vi "MainVI.vi"() -> ()   [LabVIEW 2026]
uses:
  <instrlib>/MicroPulse/Public/Data/Datatypes/TCP config.ctl
  <instrlib>/MicroPulse/Public/Data/Datatypes/MP - pulser voltage.ctl
  <instrlib>/MicroPulse/Public/Data/Datatypes/MP - pulse damping.ctl
  <instrlib>/MicroPulse/Public/Data/Datatypes/MP - frequency filter.ctl
  <instrlib>/MicroPulse/Public/Data/Datatypes/MP - waveform type.ctl
  <instrlib>/MicroPulse/Public/Data/Datatypes/MP - data output format.ctl
  <instrlib>/MicroPulse/Public/Data/Datatypes/MP - amplitude reporting mode.ctl
  <instrlib>/MicroPulse/Public/Data/Datatypes/MP - averaging.ctl
  <instrlib>/MicroPulse/Public/Data/Datatypes/MP - echo gate mode.ctl
  <instrlib>/MicroPulse/MicroPulse_Driver.lvlib
panel:
  in  "stop":bool
  in  "Tab Control":T1(tab)
  in  "Calculated Diameter":T2
  in  "Calculate Scan":bool
  in  "Scan Information":T3
  in  "Scan Settings":T4
  in  "Channel Select Tab Control":enum32{"1", "2", "3", "4", "5", "6", "7"}(tab)
  in  "Damping":T5=enum."149W"
  in  "Flaw Gate (mm Ti)":T6
  in  "Backwall Gate (mm)":T7
  in  "Voltage":T8=enum."200V"
  in  "Width (ns)":u32=80
  in  "Smoothing":u16=1 caption="Smoothing (1-11)"
  in  "Filter":T9=enum."0.75-12MHz  Broadband"
  in  "Waveform Type":T10
  in  "A-Scan Window":cluster{"Start":dbl, "Range":dbl}={"Start"=0.0, "Range"=330.0}
  in  "C-Scan Collection":T11
  in  "Channel 1 Interface":T7
  in  "Gain (dB)":dbl=30.0 min=-6.0 max=70.0 step=0.25 format="%.2fdB"
  in  "Voltage 2":T8=enum."200V" caption="Voltage"
  in  "Damping 2":T5=enum."149W"
  in  "Width (ns)      2":u32=80
  in  "Gain (dB) 2":dbl=30.0 min=-6.0 max=70.0 step=0.25 format="%.2fdB"
  in  "Filter 2":T9=enum."0.75-12MHz  Broadband" caption="Filter"
  in  "Smoothing 2":u16=1 caption="Smoothing (1-11)"
  in  "Waveform Type 2":T10 caption="Waveform Type"
  in  "A-Scan Window 2":cluster{"Start":dbl, "Range":dbl}={"Start"=0.0, "Range"=330.0}
  out "Waveform Graph":u16[](graph)
  in  "Channel Select":string(combo)="1"
  in  "PRF":u16=50
  in  "MicroPulse Configuration":T12={"Connection ID"=refnum, "IP address"="10.1.1.2", "host port"=1067, "OC timeout"=-1, "Read timeout"=0, "Write timeout"=0} {"Write timeout" format="%dms"; "Read timeout" format="%dms"; "OC timeout" format="%dms"}
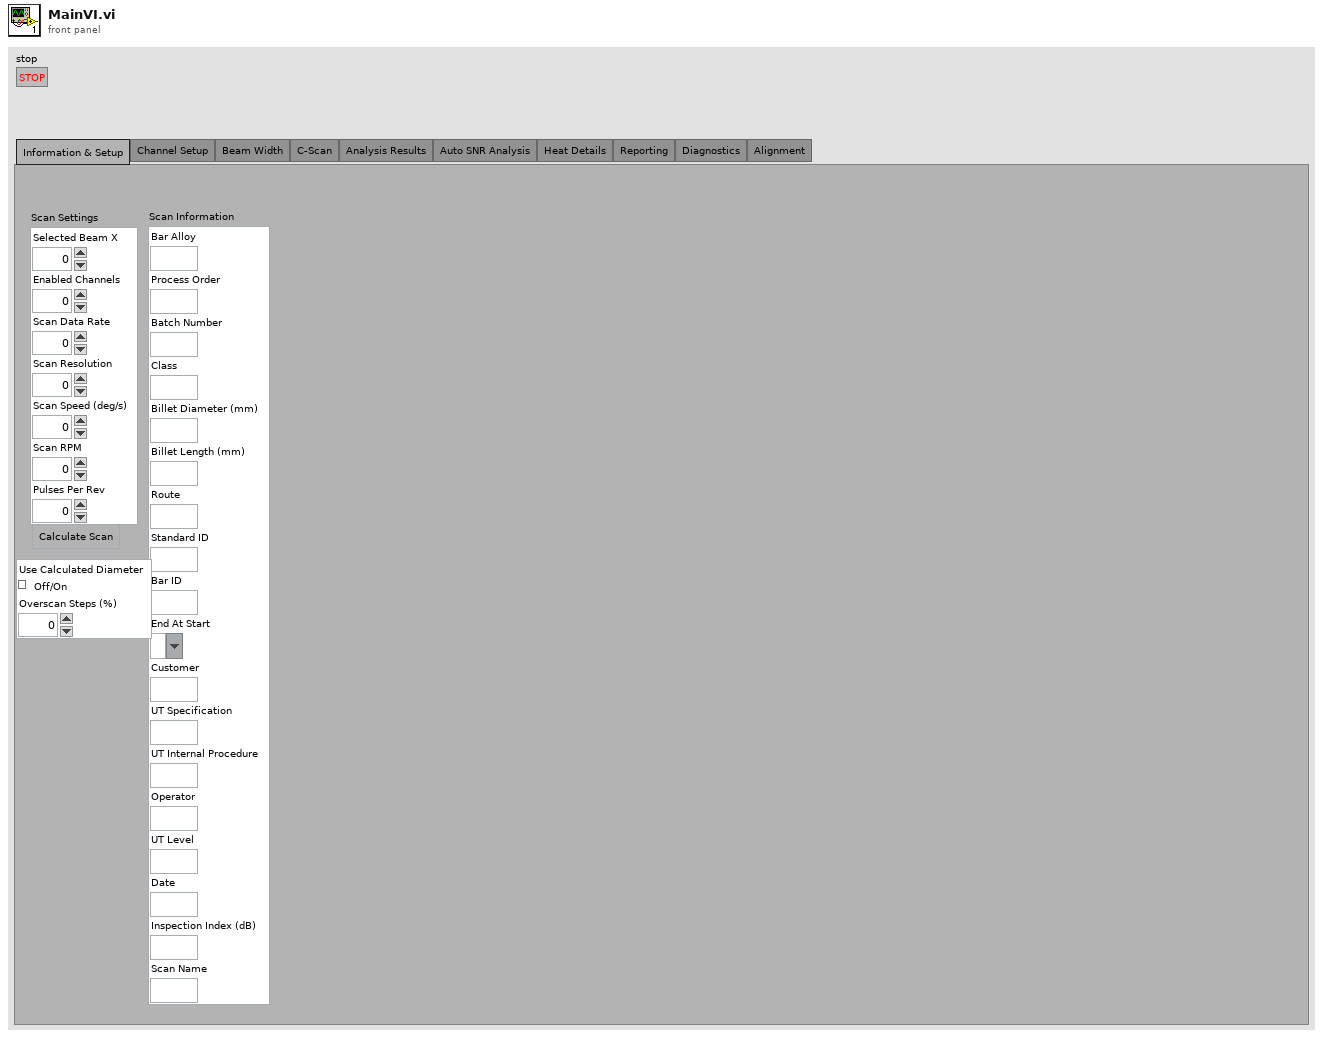
[diagram p1: front panel]
types:
  T1 = enum32{"Information & Setup", "Channel Setup", "Beam Width", "C-Scan", "Analysis Results", "Auto SNR Analysis", "Heat Details", "Reporting", "Diagnostics", "Alignment"}
  T2 = cluster{"Use Calculated Diameter":bool, "Overscan Steps (%)":dbl}
  T3 = cluster{"Bar Alloy":string, "Process Order":string, "Batch Number":string, "Class":string, "Billet Diameter (mm)":string, "Billet Length (mm)":string, "Route":string, "Standard ID":string, "Bar ID":string, "End At Start":string, "Customer":string, "UT Specification":string, "UT Internal Procedure":string, "Operator":string, "UT Level":string, "Date":string, "Inspection Index (dB)":string, "Scan Name":string}
  T4 = cluster{"Selected Beam X":dbl, "Enabled Channels":dbl, "Scan Data Rate":dbl, "Scan Resolution":dbl, "Scan Speed (deg/s)":dbl, "Scan RPM":dbl, "Pulses Per Rev":dbl}
  T5 = typedef "MicroPulse_Driver.lvlib/MP - pulse damping.ctl" = enum16{"660W", "458W", "220W", "149W", "102W", "82W", "63W", "51W"}
  T6 = cluster{"Start":dbl, "Length":dbl, "Threshold":dbl, "Water Path":dbl, "Gate Amplitude":dbl, "Gate TOF":dbl}
  T7 = cluster{"Start":dbl, "Length":dbl, "Threshold":dbl}
  T8 = typedef "MicroPulse_Driver.lvlib/MP - pulser voltage.ctl" = enum16{"50V", "100V", "150V", "200V", "250V", "300V"}
  T9 = typedef "MicroPulse_Driver.lvlib/MP - frequency filter.ctl" = enum16{"No change", "1MHz Bandpass", "2MHz Bandpass", "4MHz Bandpass", "5MHz Bandpass", "10MHz Bandpass", "2.5-18MHz Broadband", "0.75-12MHz  Broadband", "0.5MHz Bandpass", "5MHz 2nd Order TOFD", "10MHz 2nd Order TOFD", "3.0-25MHz Broadband", "3.0-30MHz Broadband"}
  T10 = typedef "MicroPulse_Driver.lvlib/MP - waveform type.ctl" = enum16{"Rectified Signal", "RF Signal", "+Half Wave", "-Half Wave"}
  T11 = cluster{"Flaw Gate Amplitude":bool, "Flaw Gate TOF":bool, "Backwall Gate Amplitude":bool, "Backwall Gate TOF":bool}
  T12 = typedef "MicroPulse_Driver.lvlib/TCP config.ctl" = cluster{"Connection ID":refnum<k5>, "IP address":string, "host port":u16, "OC timeout":i32, "Read timeout":i32, "Write timeout":i32}
  T13 = typedef "MicroPulse_Driver.lvlib/MP - data output format.ctl" = enum16{"", "8-bit Mode", "10-bit Mode", "12-bit Mode", "16-bit Mode", "8-bit Log Mode", "12-bit Packed Mode"}
  T14 = typedef "MicroPulse_Driver.lvlib/MP - echo gate mode.ctl" = enum16{"Echo Trigger OFF", "Echo Gate Display Mode", "Echo Trigger ON", "Multi Gate or FMC Mode", "Reserved", "PA - Echo Trigger ON"}
  T15 = typedef "MicroPulse_Driver.lvlib/MP - averaging.ctl" = enum16{"None", "2", "4", "8", "16", "32", "64", "128", "256"}
  T16 = typedef "MicroPulse_Driver.lvlib/MP - amplitude reporting mode.ctl" = enum16{"1st Peak in gate", "Maximum Peak in gate", "All Peaks", "Ascan Data", "1st Threshold Crossing Peak", "Ascan + Peaks", "All Peaks for Multigate", "Peaks + Ascan for Multigate", "Peaks + P_Ascan for Multigate", "Full Matrix Capture"}
  T17 = typedef "MicroPulse_Driver.lvlib/MP - scan data info.ctl" = cluster{"Message Header":u16, "Error Message":u16, "Test No.":u32, "Channel No.":u8, "Sweep No.":u32, "Gate No.":u32, "DOF":T13, "retain data":T18, "scan data":u16[], "scan length":i32, "scan index":i32, "peak data":cluster{"timebase":u16[], "data":u16[]}, "#peaks":i32, "PRF":dbl, "IP":cluster{"Axis No.":u8, "Location":u32, "MIP location":u32, "MIP?":bool}, "echo range":u16, "ETG":bool, "CAL 0 complete":bool, "Axis Positions":T19}
  T18 = typedef "MicroPulse_Driver.lvlib/MP - retain scan.ctl" = enum16{"None", "Ascan", "Peaks"}
  T19 = typedef "MicroPulse_Driver.lvlib/MP - axis positions (LLC).ctl" = cluster{"Axis 1":u32, "Axis 2":u32, "Axis 3":u32, "Axis 4":u32, "Status":u8}
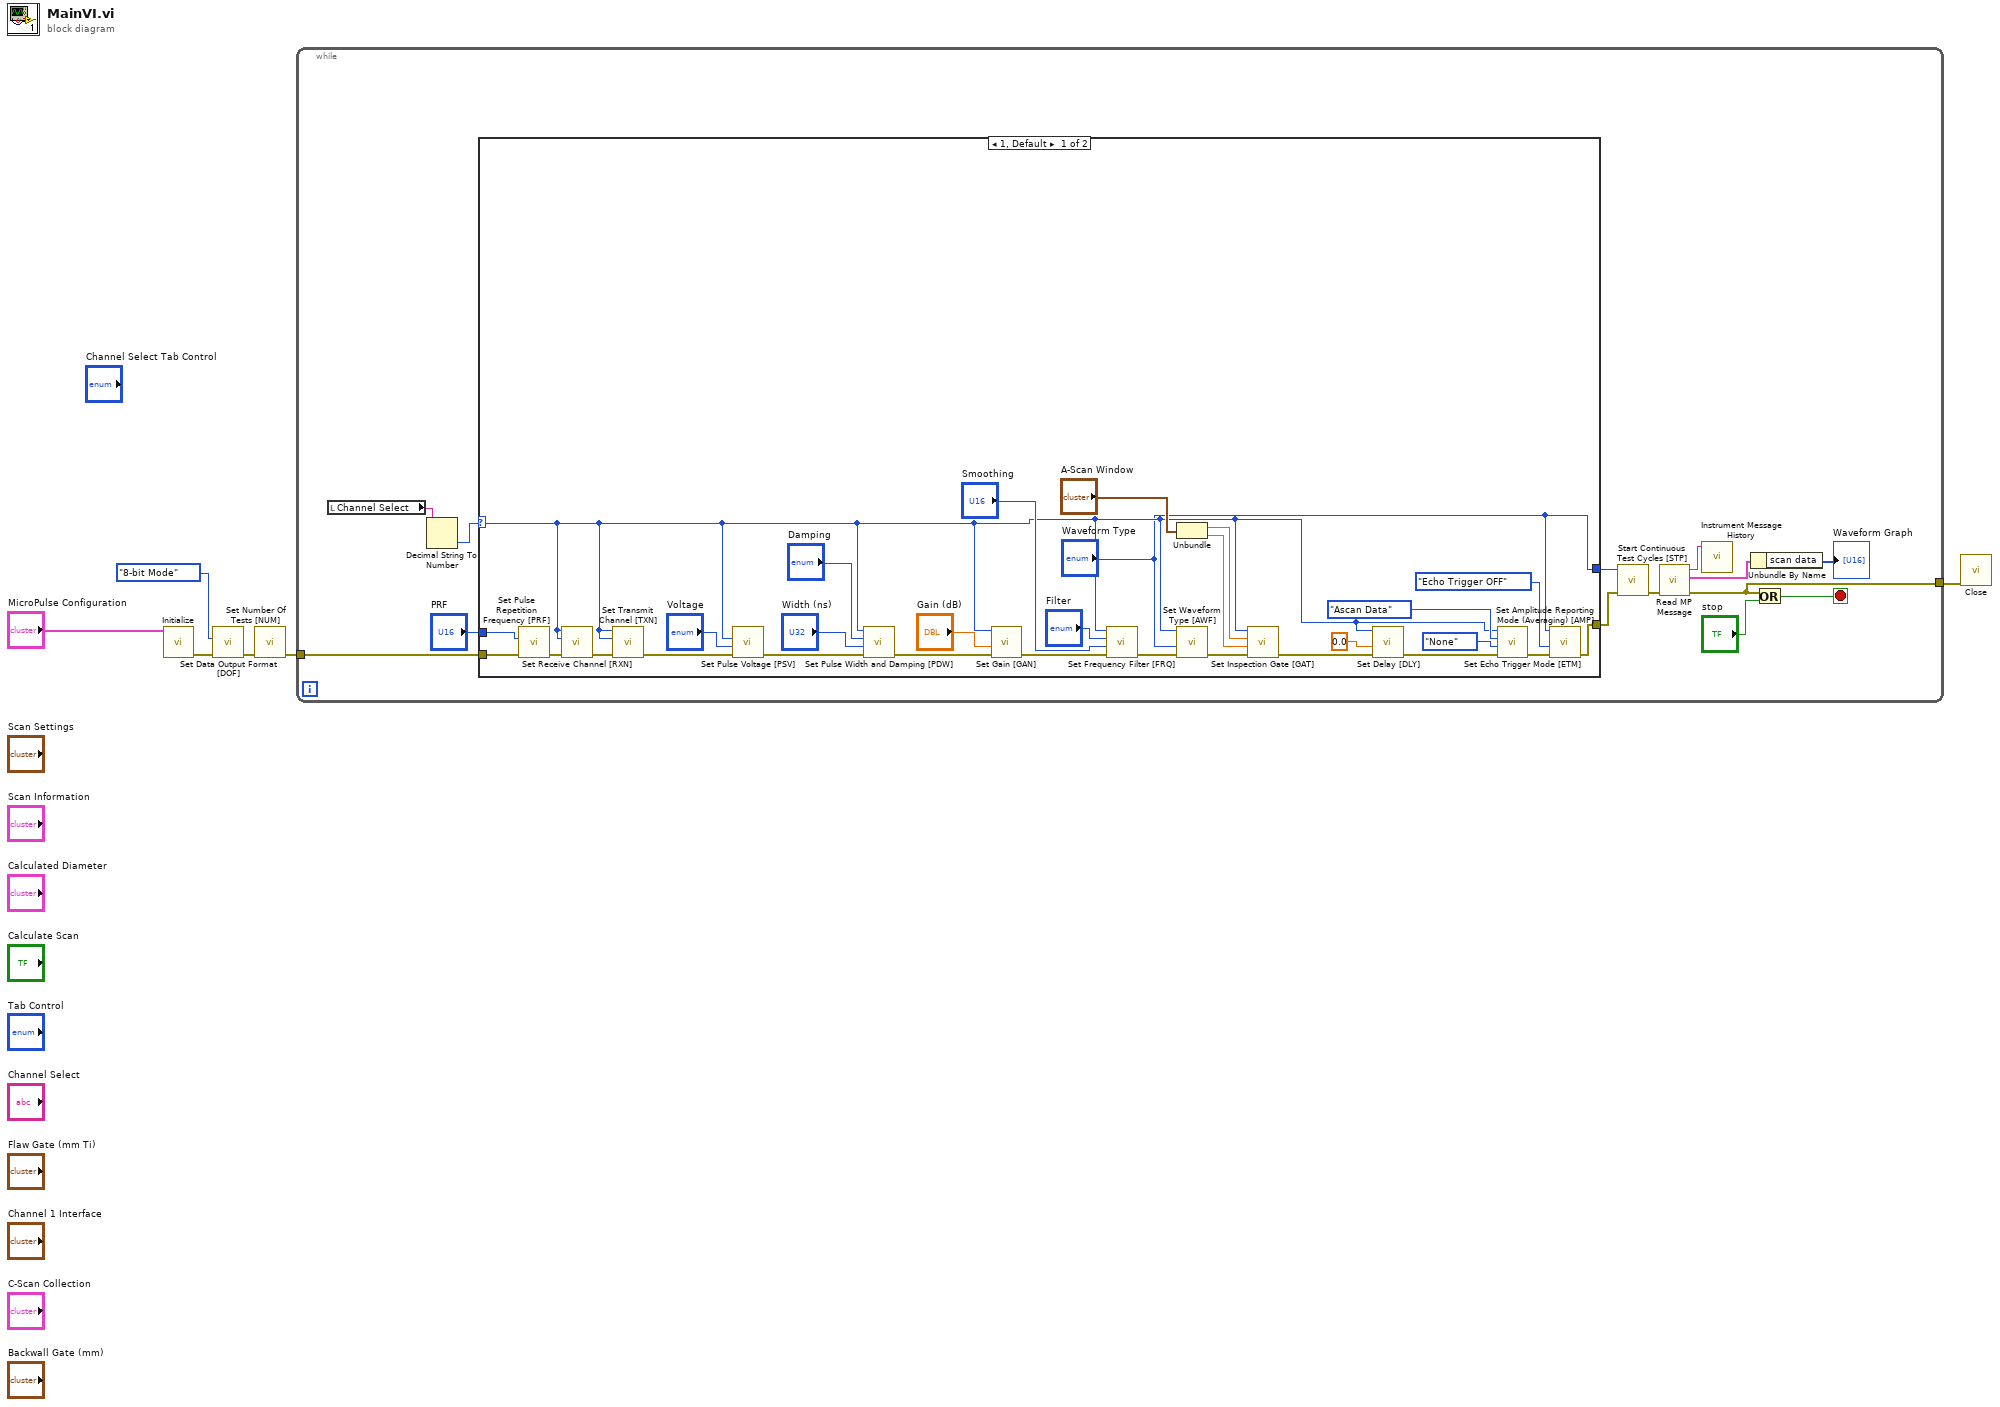
[diagram p0: block diagram]
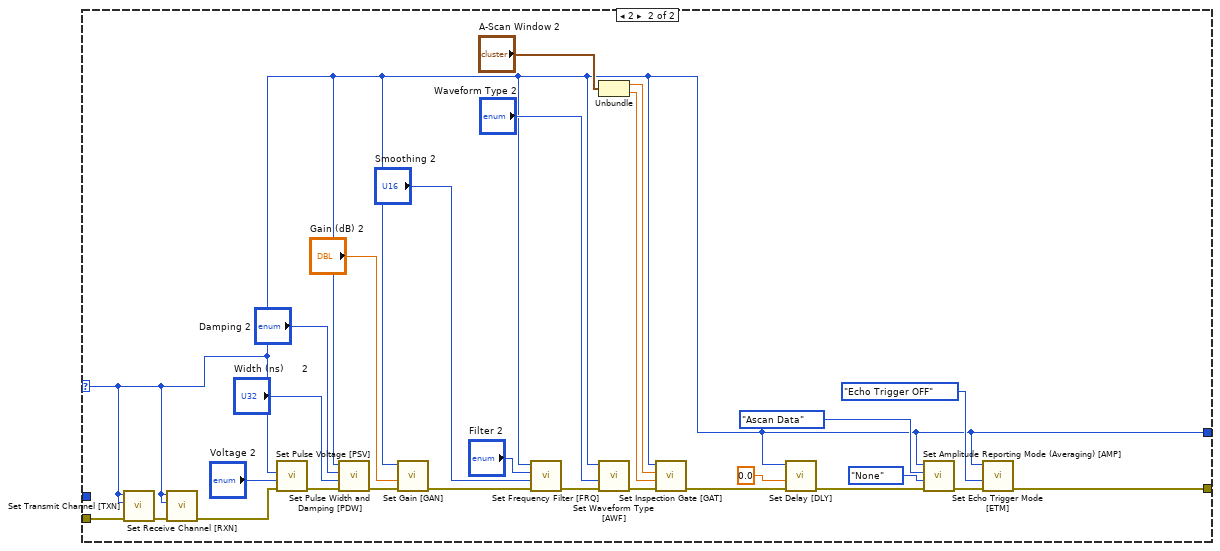
[diagram p2: hidden frame]
diagram:
  n1 = call <instrlib>:"Initialize.vi"("TCP config"="MicroPulse Configuration") -> ("error out"=w3:errorcluster)  [unwired: 9 in, 1 out]
  n2 = call "Set Data Output Format [DOF].vi"("error in (no error)"=w3, "Mode"=MP_-_data_output_format."8-bit Mode") -> ("error out"=w5:errorcluster)  [unwired: 8 in, 1 out]
  n3 = call <instrlib>:"Set Number Of Tests [NUM].vi"("error in (no error)"=w5) -> ("error out"=w2:errorcluster)  [unwired: 8 in, 2 out]
  n4 = while {
    tunnel: w2 -> [w16]
    tunnel: [w11] -> w1
    stop <- w12 stop-if-true
    n5 = local read "Channel Select"() -> (w8:string)
    n6 = Decimal String To Number(string=w8) -> (number=w7:i32)  [unwired: 2 in, 1 out]
    n7 = case shown="1, Default" w7 {
      selector: w7 -> [w25 w49]
      tunnel: w16 -> [w22 w61]
      tunnel: ["Waveform Type" w49] -> w14
      tunnel: [w20 w50] -> w9
      tunnel: "PRF" -> [w23 _]
      frame 1, Default {
        n8 = call <instrlib>:"Set Pulse Repetition Frequency [PRF].vi"("error in (no error)"=w22, "Frequency (Hz)"=w23) -> ("error out"=w21:errorcluster)  [unwired: 8 in, 1 out]
        n9 = call <instrlib>:"Set Receive Channel [RXN].vi"("error in (no error)"=w21, "Channel Number"=w25, "Test Number"=w25) -> ("error out"=w35:errorcluster)  [unwired: 7 in, 1 out]
        n10 = call <instrlib>:"Set Transmit Channel [TXN].vi"("error in (no error)"=w35, "Channel Number"=w25, "Test Number"=w25) -> ("error out"=w34:errorcluster)  [unwired: 7 in, 1 out]
        n11 = call <instrlib>:"Set Pulse Voltage [PSV].vi"("error in (no error)"=w34, "Voltage"="Voltage", "Channel Number"=w25) -> ("error out"=w33:errorcluster)  [unwired: 7 in, 1 out]
        n12 = call <instrlib>:"Set Pulse Width and Damping [PDW].vi"("error in (no error)"=w33, "Width (ns)"="Width (ns)", "Damping"="Damping", "Channel Number"=w25) -> ("error out"=w32:errorcluster)  [unwired: 6 in, 1 out]
        n13 = call <instrlib>:"Set Gain [GAN].vi"("error in (no error)"=w32, "Gain (dB)"="Gain (dB)", "Test Number"=w25) -> ("error out"=w31:errorcluster)  [unwired: 7 in, 1 out]
        n14 = call <instrlib>:"Set Frequency Filter [FRQ].vi"("error in (no error)"=w31, "Smoothing"="Smoothing", "Filter"="Filter", "Test Number"=w25) -> ("error out"=w30:errorcluster)  [unwired: 6 in, 1 out]
        n15 = Unbundle("A-Scan Window") -> ("Start"=w41:dbl, "Range"=w40:dbl)
        n16 = call <instrlib>:"Set Waveform Type [AWF].vi"("error in (no error)"=w30, "Waveform Type"="Waveform Type", "Test Number"=w25) -> ("error out"=w29:errorcluster)  [unwired: 7 in, 1 out]
        n17 = call <instrlib>:"Set Inspection Gate [GAT].vi"("error in (no error)"=w29, "Gate Length (us)"=w40, "Gate Start (us)"=w41, "Test Number"=w25) -> ("error out"=w28:errorcluster)  [unwired: 6 in, 1 out]
        n18 = call <instrlib>:"Set Delay [DLY].vi"("error in (no error)"=w28, "Delay (us)"=0.0, "Test Number"=w25) -> ("error out"=w27:errorcluster)  [unwired: 7 in, 1 out]
        n19 = call <instrlib>:"Set Amplitude Reporting Mode (Averaging) [AMP].vi"("error in (no error)"=w27, "Averaging"=MP_-_averaging."None", "Amplitude Mode"=MP_-_amplitude_reporting_mode."Ascan Data", "Test Number"=w25) -> ("error out"=w26:errorcluster)  [unwired: 6 in, 1 out]
        n20 = call <instrlib>:"Set Echo Trigger Mode [ETM].vi"("error in (no error)"=w26, "ETM Mode"=MP_-_echo_gate_mode."Echo Trigger OFF", "Test Number"="Waveform Type") -> ("error out"=w20:errorcluster)  [unwired: 7 in, 1 out]
      }
      frame 2 {
        n21 = call <instrlib>:"Set Transmit Channel [TXN].vi"("error in (no error)"=w61, "Channel Number"=w49, "Test Number"=w49) -> ("error out"=w60:errorcluster)  [unwired: 7 in, 1 out]
        n22 = call <instrlib>:"Set Receive Channel [RXN].vi"("error in (no error)"=w60, "Channel Number"=w49, "Test Number"=w49) -> ("error out"=w59:errorcluster)  [unwired: 7 in, 1 out]
        n23 = call <instrlib>:"Set Pulse Voltage [PSV].vi"("error in (no error)"=w59, "Voltage"="Voltage 2", "Channel Number"=w49) -> ("error out"=w58:errorcluster)  [unwired: 7 in, 1 out]
        n24 = call <instrlib>:"Set Pulse Width and Damping [PDW].vi"("error in (no error)"=w58, "Width (ns)"="Width (ns)      2", "Damping"="Damping 2", "Channel Number"=w49) -> ("error out"=w57:errorcluster)  [unwired: 6 in, 1 out]
        n25 = call <instrlib>:"Set Gain [GAN].vi"("error in (no error)"=w57, "Gain (dB)"="Gain (dB) 2", "Test Number"=w49) -> ("error out"=w56:errorcluster)  [unwired: 7 in, 1 out]
        n26 = call <instrlib>:"Set Frequency Filter [FRQ].vi"("error in (no error)"=w56, "Smoothing"="Smoothing 2", "Filter"="Filter 2", "Test Number"=w49) -> ("error out"=w55:errorcluster)  [unwired: 6 in, 1 out]
        n27 = Unbundle("A-Scan Window 2") -> ("Start"=w67:dbl, "Range"=w66:dbl)
        n28 = call <instrlib>:"Set Waveform Type [AWF].vi"("error in (no error)"=w55, "Waveform Type"="Waveform Type 2", "Test Number"=w49) -> ("error out"=w54:errorcluster)  [unwired: 7 in, 1 out]
        n29 = call <instrlib>:"Set Inspection Gate [GAT].vi"("error in (no error)"=w54, "Gate Length (us)"=w66, "Gate Start (us)"=w67, "Test Number"=w49) -> ("error out"=w53:errorcluster)  [unwired: 6 in, 1 out]
        n30 = call <instrlib>:"Set Delay [DLY].vi"("error in (no error)"=w53, "Delay (us)"=0.0, "Test Number"=w49) -> ("error out"=w52:errorcluster)  [unwired: 7 in, 1 out]
        n31 = call <instrlib>:"Set Amplitude Reporting Mode (Averaging) [AMP].vi"("error in (no error)"=w52, "Averaging"=MP_-_averaging."None", "Amplitude Mode"=MP_-_amplitude_reporting_mode."Ascan Data", "Test Number"=w49) -> ("error out"=w51:errorcluster)  [unwired: 6 in, 1 out]
        n32 = call <instrlib>:"Set Echo Trigger Mode [ETM].vi"("error in (no error)"=w51, "ETM Mode"=MP_-_echo_gate_mode."Echo Trigger OFF", "Test Number"=w49) -> ("error out"=w50:errorcluster)  [unwired: 7 in, 1 out]
      }
    }
    n33 = call <instrlib>:"Start Continuous Test Cycles [STP].vi"("error in (no error)"=w9, "Test Number"=w14) -> ("error out"=w15:errorcluster)  [unwired: 8 in, 1 out]
    n34 = call <instrlib>:"Read MP Message.vi"("error in (no error)"=w15) -> ("error out"=w11:errorcluster, "scan data info"=w18:T17, "Instrument Message"=w19:string)  [unwired: 6 in, 2 out]
    n35 = call <instrlib>:"Instrument Message History.vi"("Instrument Message"=w19) -> ()  [unwired: 9 in, 2 out]
    n36 = Unbundle By Name(w18) -> ("scan data"=→"Waveform Graph":u16[])
    n37 = Or(x=w11, y="stop") -> (x .or. y?=w12:bool)
  }
  n38 = call <instrlib>:"Close.vi"("error in (no error)"=w1) -> ()  [unwired: 9 in, 2 out]
